vi "Read U32.vi"(8 "error in":errorcluster, 9 "RegisterOffset":u32, 10 "register name":string, 11 "session in":u32) -> (0 "error out":errorcluster, 2 "value out":u32, 3 "session out":u32)   [LabVIEW 2020, in "FPGA Register IO.lvlib"]
uses:
  FPGA Register IO.lvlib
  NiFpga.dll
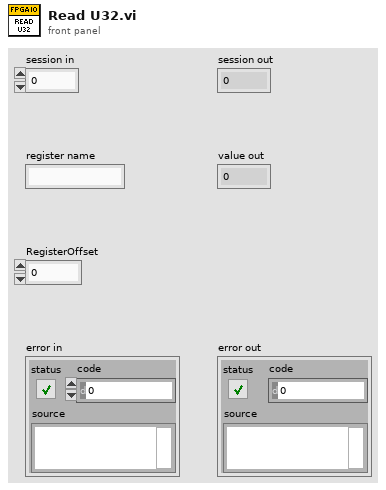
[diagram p1: front panel]
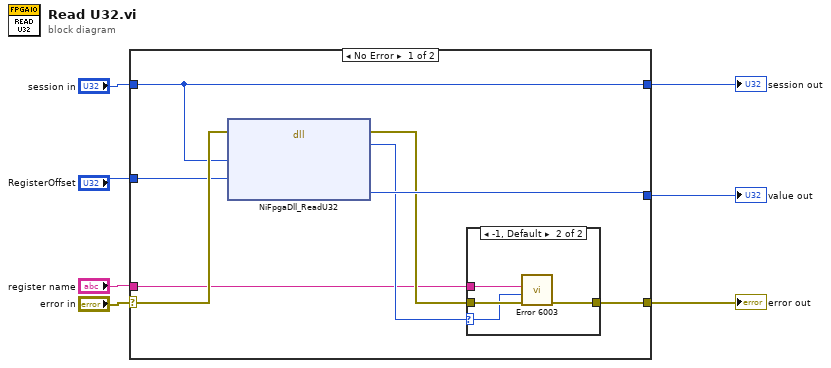
[diagram p0: block diagram]
diagram:
  n1 = case shown="No Error" "error in" {
    selector: "error in" -> [w14 w22]
    tunnel: "session in" -> [w13 w21]
    tunnel: [w10 w22] -> w7
    tunnel: [w15 _] -> w6
    tunnel: [w13 w21] -> w5
    tunnel: "RegisterOffset" -> [w12 _]
    tunnel: "register name" -> [w8 _]
    frame No Error {
      n2 = dll-call lib="NiFpga.*" fn="NiFpgaDll_ReadU32"(error in=w14, "session"=w13, "offset"=w12) -> (error out=w11:errorcluster, "status"=w9:i32, "value"=w15:u32)  [unwired: 5 in, 1 out]
      n3 = case shown="-1, Default" w9 {
        selector: w9 -> [_ w17]
        tunnel: w11 -> [w16 w20]
        tunnel: [w16 w19] -> w10
        tunnel: w8 -> [_ w18]
        frame 0 {
        }
        frame -1, Default {
          n4 = call "Error 6003.vi"("error in (no error)"=w20, "rio status code"=w17, "register name"=w18) -> ("error out"=w19:errorcluster)  [unwired: 8 in]
        }
      }
    }
    frame Error {
    }
  }
  "error out" <- w7
  "session out" <- w5
  "value out" <- w6
